vi "SysCfgTest.vi"() -> ()   [LabVIEW 2020]
uses:
  <vilib>/nisyscfg/Close (Hardware).vi
  <vilib>/nisyscfg/Close (System).vi
  <vilib>/nisyscfg/nisyscfg.lvlib
  <resource>/objmgr/niMIDebugSession.rc
panel:
  in  "IVI Logical Name":refnum<k15>
  out "Detailed Result":string
  out "error out":errorcluster
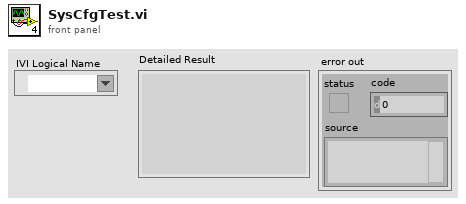
[diagram p1: front panel]
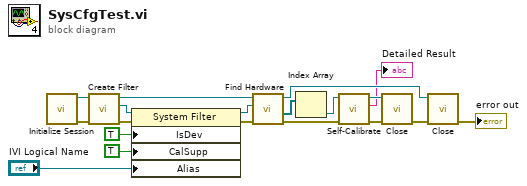
[diagram p0: block diagram]
diagram:
  n1 = call <vilib>:"Initialize Session.vi"() -> ("error out"=w14:errorcluster, "Session out"=w15:refnum<k21>)  [unwired: 10 in]
  n2 = call <vilib>:"Create Filter.vi"("error in (no error)"=w14, "Session in"=w15) -> ("error out"=w17:errorcluster, "Filter out"=w16:refnum<k20>, "Session out"=w11:refnum<k21>)  [unwired: 7 in]
  n3 = property class="System Filter"(reference=w16, error in=w17, "IsDev"=TRUE ("Is Device"), "CalSupp"=TRUE ("Devices & Chassis:Supports Calibration"), "Alias"="IVI Logical Name") -> (reference out=w12:refnum<k20>, error out=w13:errorcluster)
  n4 = call <vilib>:"Find Hardware.vi"("error in (no error)"=w13, "Filter in"=w12, "Session in"=w11) -> ("error out"=w7:errorcluster, "Resources out"=w8:refnum<k20>[], "Session out"=w19:refnum<k21>)  [unwired: 5 in, 1 out]
  n5 = Index Array(array=w8) -> (element=w5:refnum<k20>)  [unwired: 1 in]
  n6 = call <vilib>:"Self-Calibrate.vi"("error in (no error)"=w7, "Resource in"=w5) -> ("error out"=w6:errorcluster, "Detailed Result"=→"Detailed Result":string, "Resource out"=w4:refnum<k20>)  [unwired: 7 in]
  n7 = call-poly <vilib>:"Close.vi"("error in (no error)"=w6, "Resource in"=w4) -> ("error out"=w2:errorcluster)  [unwired: 9 in]
  n8 = call-poly <vilib>:"Close.vi"("error in (no error)"=w2, "Session in"=w19) -> ("error out"=→"error out":errorcluster)  [unwired: 9 in]
